vi "Python@GetPoint(Worker)__Parameter.vi"(1 "ParamterIn":string) -> (0 "ParamterOut":string)   [LabVIEW 2020]
panel:
  in  "Session":string(combo)
  in  "ARCOSName":string(combo) caption="ARCOSName="
  in  "PythonVariable":string(combo)
  in  "Confirm":bool
  # "Python@GetPoint(Worker) $Worker,$PythonPoint(,ARCOSName=)"
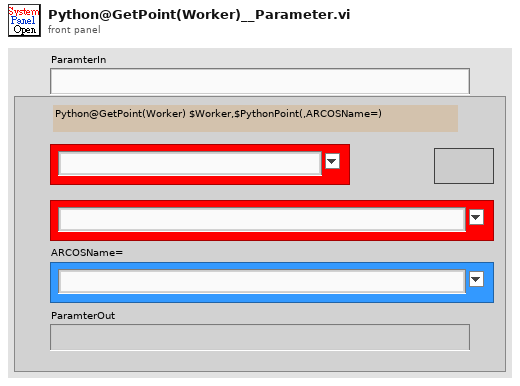
[diagram p1: front panel]
types:
  T1 = enum16{"Get", "UpdatePointS", "Init", "UpdateIndex", "GetCurrent&Index+1", "GetWithIndex", "ChkLast", "GetCurrent"}
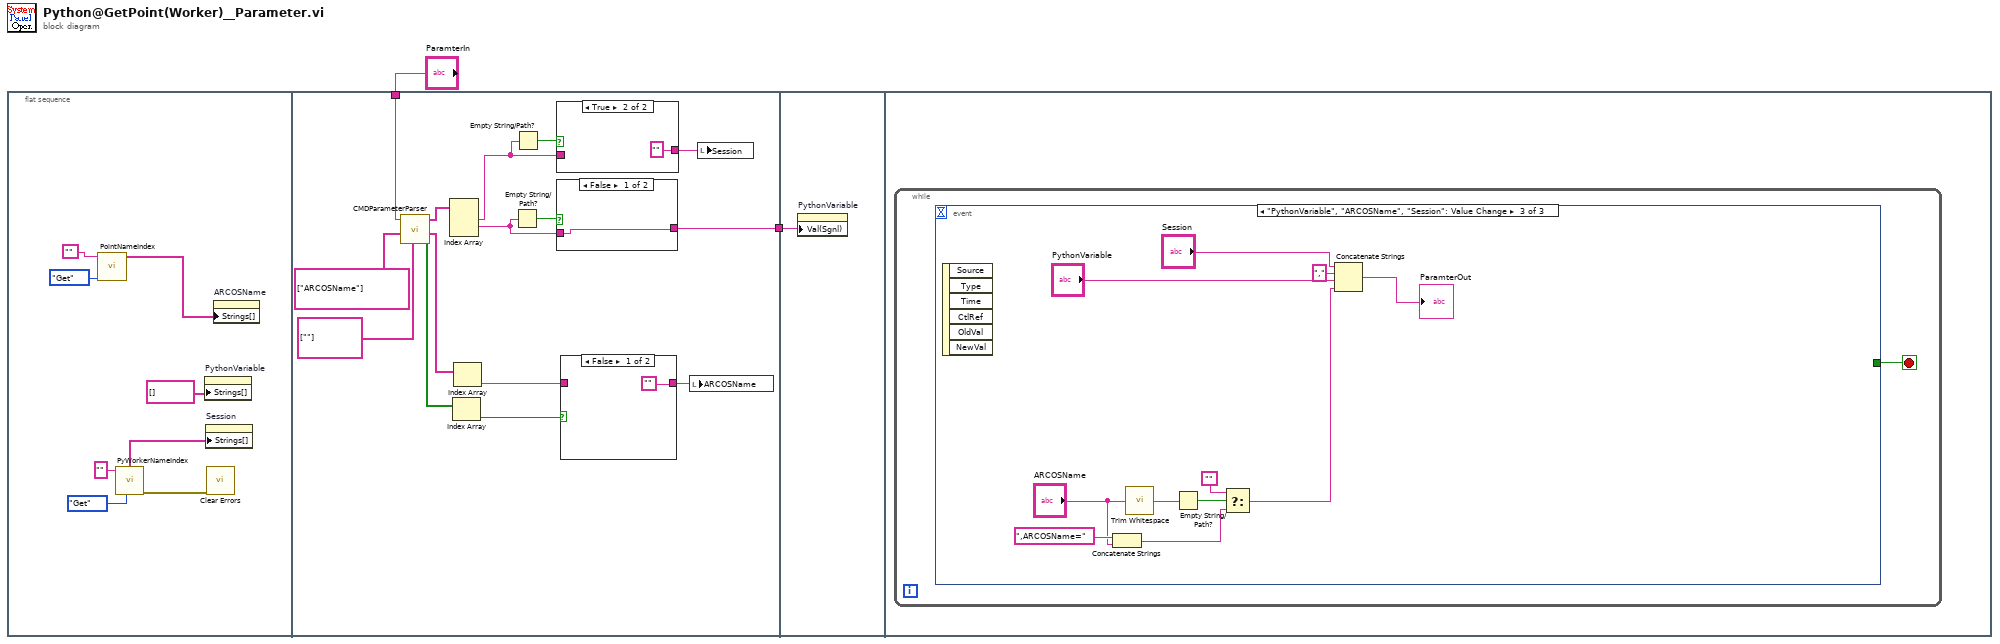
[diagram p0: block diagram]
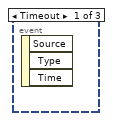
[diagram p5: hidden frame]
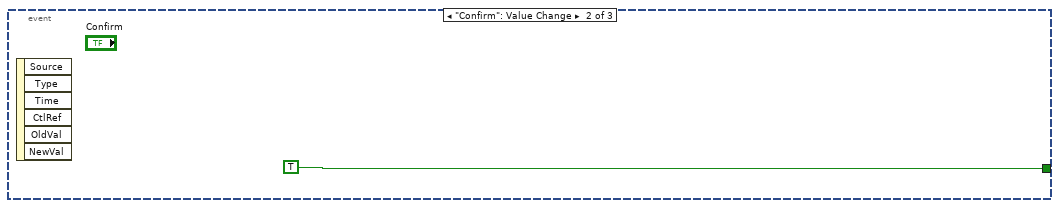
[diagram p6: hidden frame]
diagram:
  n1 = flat-sequence {
    tunnel: "ParamterIn" -> [w22]
    tunnel: [w24] -> w1
    tunnel: w1 -> [w32]
    frame #0 {
      n2 = call "PointNameIndex.vi"("OP"=T1."Get", "PointName"="") -> ("PointNameList"=w7:string[])  [unwired: 4 in, 5 out]
      n3 = call "PyWorkerNameIndex.vi"("OP"=enum16{"Init", "Get", "Set"}."Get", "WrokerName"="" ("SessionIn")) -> ("error out"=w3:errorcluster, "PythonWorkerNameS"=w4:string[])  [unwired: 6 in, 2 out]
      n4 = property on="PythonVariable" class="CmbBox"("Strings[]"=string[] [] ("Strings []")) -> ()  [unwired: 2 in, 2 out]
      n5 = property on="Session" class="CmbBox"("Strings[]"=w4) -> ()  [unwired: 2 in, 2 out]
      n6 = call <vilib>:"Clear Errors.vi"("error in (no error)"=w3) -> ()  [unwired: 5 in, 2 out]
      n7 = property on="ARCOSName" class="CmbBox"("Strings[]"=w7) -> ()  [unwired: 2 in, 2 out]
    }
    frame #1 {
      n8 = call "CMDParameterParser.vi"("DeafultValues"=string[] [""], "RequiredKeys"=string[] ["ARCOSName"], "CMDParameter"=w22) -> ("KeyFind?"=w17:bool[], "KeyValues"=w18:string[], "Input"=w21:string[])  [unwired: 6 in]
      n9 = Index Array(array=w21) -> (element #1=w12:string, element #2=w23:string)  [unwired: 3 in, 1 out]
      n10 = Index Array(array=w17) -> (element=w16:bool)  [unwired: 1 in]
      n11 = Index Array(array=w18) -> (element=w15:string)  [unwired: 1 in]
      n12 = Empty String/Path?(string/path=w23) -> (empty?=w25:bool)
      n13 = Empty String/Path?(string/path=w12) -> (empty?=w13:bool)
      n14 = case shown="False" w25 {
        tunnel: w23 -> [w30 w31]
        tunnel: [w30 w31] -> w24
        frame False {
        }
        frame True {
        }
      }
      n15 = case shown="True" w13 {
        tunnel: w12 -> [w26 _]
        tunnel: [w26 ""] -> w11
        frame False {
        }
        frame True {
        }
      }
      n16 = case shown="False" w16 {
        tunnel: w15 -> [_ w29]
        tunnel: ["" w29] -> w14
        frame False {
        }
        frame True {
        }
      }
      n17 = local write "ARCOSName"(w14) -> ()
      n18 = local write "Session"(w11) -> ()
    }
    frame #2 {
      n19 = property on="PythonVariable" class="CmbBox"("Val(Sgnl)"=w32) -> ()  [unwired: 2 in, 2 out]
    }
    frame #3 {
      n20 = while {
        stop <- w33 stop-if-true
        n21 = event shown="[2] \"PythonVariable\", \"ARCOSName\", \"Session\": Value Change" {
          selector: _ -> [_ _ _]
          dyn-events: _ -> [_ _ _]
          timeout: _ -> [_ _ _]
          tunnel: [_ TRUE _] -> w33
          event Timeout {
            n22 = event-data() -> ()  [unwired: 1 in, 3 out]
          }
          event "Confirm": Value Change {
            n23 = event-data() -> ()  [unwired: 1 in, 6 out]
          }
          event "PythonVariable", "ARCOSName", "Session": Value Change {
            n24 = event-data() -> ()  [unwired: 1 in, 6 out]
            n25 = Concatenate Strings(",ARCOSName=" ("string"), "ARCOSName") -> (w38:string)
            n26 = call <vilib>:"Trim Whitespace.vi"("string"="ARCOSName") -> ("trimmed string"=w41:string)  [unwired: 1 in]
            n27 = Empty String/Path?(string/path=w41) -> (empty?=w40:bool)
            n28 = Select(t="", s=w40, f=w38) -> (s? t:f=w37:string)
            n29 = Concatenate Strings("Session", "," ("string"), "PythonVariable", w37) -> (→"ParamterOut":string)
          }
        }
      }
    }
  }
